vi "Update AO Registers.vi"(8 "error in (no error)":errorcluster, 10 "Offset":dbl, 11 "Data in":T1) -> (0 "error out":errorcluster)   [LabVIEW 2017, in "Test Bench.lvlib"]
uses:
  Test Bench.lvlib
  Scan Engine Variables.ctl
  <instrlib>/_niInstr/FIFO Register Bus/v1/Host/niInstr FIFO Register Bus v1 Host.lvclass
  C:/Program Files (x86)/National Instruments/LabVIEW 2017/instr.lib/_niInstr/Instruction Framework/v1/Host/Instruction Target/niInstr Instruction Target v1 Host.lvclass
  <instrlib>/_niInstr/Instruction Framework/v1/Host/Instruction Framework Context/niInstr Instruction Framework Context v1 Host.lvclass
  <instrlib>/_niInstr/Instruction Framework/v1/Host/Instruction Target/niInstr Instruction Target v1 Host.lvclass
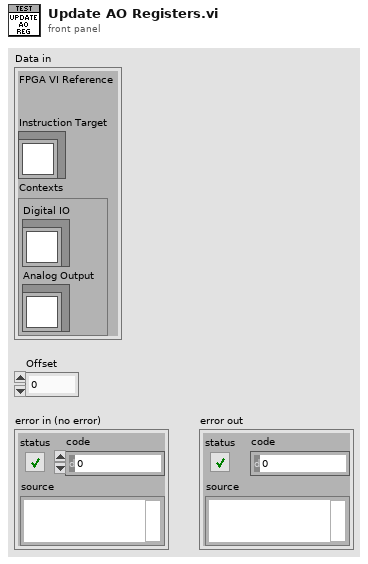
[diagram p1: front panel]
types:
  T1 = typedef "Test Bench.lvlib/Scan Engine Variables.ctl" = cluster{"FPGA VI Reference":refnum<k20>, "Instruction Target":refnum<class "niInstr FIFO Register Bus v1 Host.lvclass">, "Contexts":cluster{"Digital IO":refnum<class "niInstr Instruction Framework Context v1 Host.lvclass">, "Analog Output":refnum<class "niInstr Instruction Framework Context v1 Host.lvclass">}}
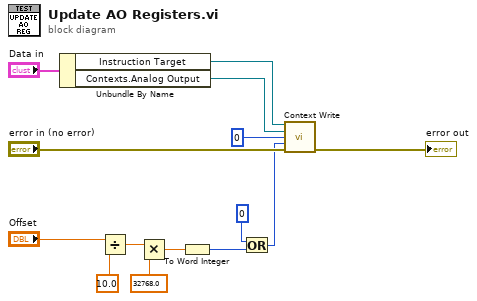
[diagram p0: block diagram]
diagram:
  n1 = Unbundle By Name("Data in") -> ("Instruction Target"=w12:refnum<class "niInstr FIFO Register Bus v1 Host.lvclass">, "Contexts.Analog Output"=w11:refnum<class "niInstr Instruction Framework Context v1 Host.lvclass">)
  n2 = Divide(x="Offset", y=10.0) -> (x/y=w6:dbl)
  n3 = Multiply(x=w6, y=32768.0) -> (x*y=w4:dbl)
  n4 = To Word Integer(number=w4) -> (16bit integer=w1:i16)
  n5 = Or(x=u64 0 ("16bit integer"), y=w1) -> (x .or. y?=w2:u64)
  n6 = call <instrlib>:"Context Write.vi"("instruction target in"=w12, "context in"=w11, "address"=u64 0, "data"=w2, "error in"="error in (no error)") -> ("error out"=→"error out":errorcluster)  [unwired: 8 in, 2 out]
